vi "Read Mixed Audio Data Queue.vi"(8 "error in (no error)":errorcluster, 11 "Mixer in":refnum<class "Mixer.lvclass">) -> (0 "error out":errorcluster, 2 "Mixed Audio Data":refnum<queue>, 3 "Mixer out":refnum<class "Mixer.lvclass">)   [LabVIEW 2020, in "G-Audio.lvlib" / "Mixer.lvclass"]
doc: "Reads the mixer audio queue. The queue is updated with a copy of the mixed audio data, which can be dequeued and used as required."
uses:
  Mixer.lvclass
  Mixer.lvclass/Mixer.ctl
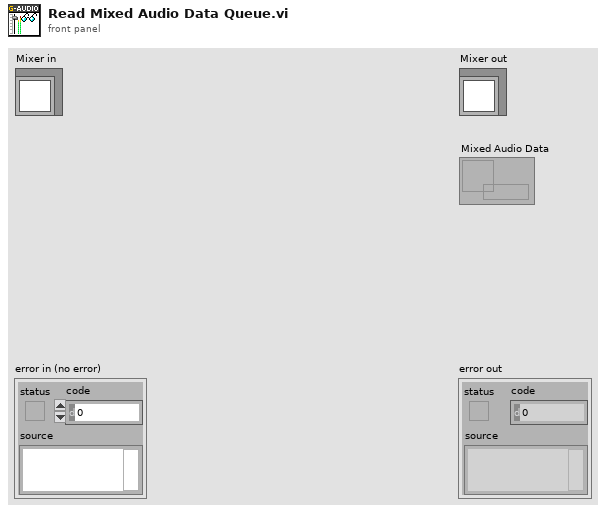
[diagram p1: front panel]
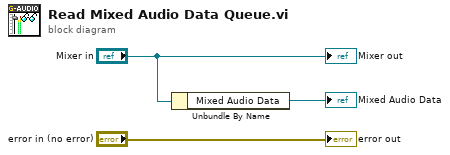
[diagram p0: block diagram]
diagram:
  n1 = Unbundle By Name("Mixer in") -> ("Mixed Audio Data"=→"Mixed Audio Data":refnum<queue>)
  "error out" <- "error in (no error)"
  "Mixer out" <- "Mixer in"
